vi "Arm Encoder.vi"(6 "Reset Encoder?":bool, 8 "Mode":enum16{"Init", "Run", "End"}(ring), 11 "Digital Module A":T1={"DIO Module"=enum."Digital Module 2", "Left Encoder B Channel"=enum."DIO 1", "Left Encoder A Channel"=enum."DIO 2", "Right Encoder B Channel"=enum."DIO 3", "Right Encoder A Channel"=enum."DIO 4", "Arm Encoder A Channel"=enum."DIO 5", "Arm Encoder B Channel"=enum."DIO 6", "Pressure Switch"=enum."DIO 7", "Unassigned"=enum."DIO 8", "Unassigned"=enum."DIO 9", "Ultrasonic Trigger"=enum."DIO 10", "Remus Switch"=enum."DIO 11", "Unassigned"=enum."DIO 12", "Unassigned"=enum."DIO 13", "Unassigned"=enum."DIO 14"}) -> (2 "Get Arm Encoder":dbl)   [LabVIEW 2013]
doc: "This example shows how to move a motor connected to an encoder and a wheel, and then read information about the system from an encoder.\n\nThis is an example of how to use feedback (from the encoder) to create an open loop system. If some control method was used, for example using PID, a closed loop system could be created."
uses:
  <vilib>/Rock Robotics/WPI/Encoder/WPI_EncoderType.ctl
  Type Defs/Digital Module A.ctl
  <vilib>/Rock Robotics/SystemInterfaces/Typedef/FPGA_TypedefDigitalModule.ctl
  <vilib>/Rock Robotics/SystemInterfaces/DIO/FPGA_DIOChannel.ctl
  <vilib>/Rock Robotics/WPI/Counter/WPI_CounterDigitalInputToDigitalSource.vi
panel:
  out "Arm Encoder Direction":string="Backward"
  in  "Decoding Type":T4=enum."4x"
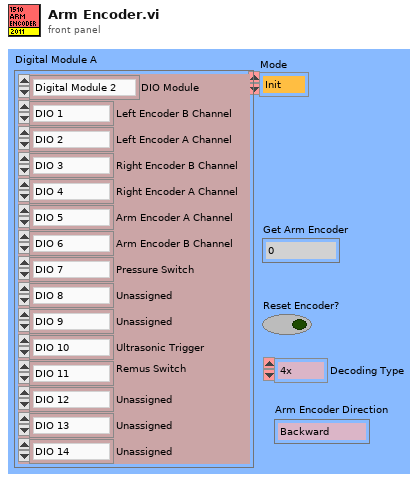
[diagram p1: front panel]
types:
  T1 = typedef "Digital Module A.ctl" = cluster{"DIO Module":T2, "Left Encoder B Channel":T3, "Left Encoder A Channel":T3, "Right Encoder B Channel":T3, "Right Encoder A Channel":T3, "Arm Encoder A Channel":T3, "Arm Encoder B Channel":T3, "Pressure Switch":T3, "Unassigned":T3, "Unassigned":T3, "Ultrasonic Trigger":T3, "Remus Switch":T3, "Unassigned":T3, "Unassigned":T3, "Unassigned":T3}
  T2 = typedef "FPGA_TypedefDigitalModule.ctl" = enum16{"Digital Module 1", "Digital Module 2"}
  T3 = typedef "FPGA_DIOChannel.ctl" = enum8{"DIO 1", "DIO 2", "DIO 3", "DIO 4", "DIO 5", "DIO 6", "DIO 7", "DIO 8", "DIO 9", "DIO 10", "DIO 11", "DIO 12", "DIO 13", "DIO 14", "Invalid"}
  T4 = typedef "WPI_EncoderType.ctl" = enum16{"1x", "2x", "4x"}
  T5 = typedef "WPI_DigitalInputDevRef.ctl" = cluster{"DevStatus":errorcluster, "DIO Channel":T3, "Digital Module":T2}
  T6 = typedef "FPGA_CounterEncoderSourceConvertionLVSourceType.ctl" = cluster{"DevStatus":errorcluster, "AnalogTriggerMode?":bool, "DigitalMode":cluster{"Digital Module":T2, "DIO Channel":T7}, "AnalogTriggerMode":cluster{"AnalogTriggerIndex":T8, "OutputType":T9}}
  T7 = typedef "FPGA_DIODigitalSourceChannel.ctl" = enum8{"DIO 1", "DIO 2", "DIO 3", "DIO 4", "DIO 5", "DIO 6", "DIO 7", "DIO 8", "DIO 9", "DIO 10", "DIO 11", "DIO 12", "DIO 13", "DIO 14", "Disabled"}
  T8 = typedef "FPGA_AnalogTriggerIndex.ctl" = enum8{"Trig 0", "Trig 1", "Trig 2", "Trig 3", "Trig 4", "Trig 5", "Trig 6", "Trig 7", "Invalid"}
  T9 = typedef "FPGA_AnalogTriggerOutType.ctl" = enum16{"InWindow", "TriggerState", "Rising", "Falling"}
  T10 = typedef "WPI_EncoderDevRef.ctl" = cluster{"DevStatus":errorcluster, "EncoderIndex":T11, "CounterIndex":T12, "DistancePerCount":dbl, "Decoding Type":T4}
  T11 = typedef "FPGA_EncoderIdx.ctl" = enum8{"Enc 0", "Enc 1", "Enc 2", "Enc 3", "Invalid"}
  T12 = typedef "FPGA_CounterCtrSystemIndex.ctl" = enum8{"Ctr 0", "Ctr 1", "Ctr 2", "Ctr 3", "Ctr 4", "Ctr 5", "Ctr 6", "Ctr 7", "Invalid"}
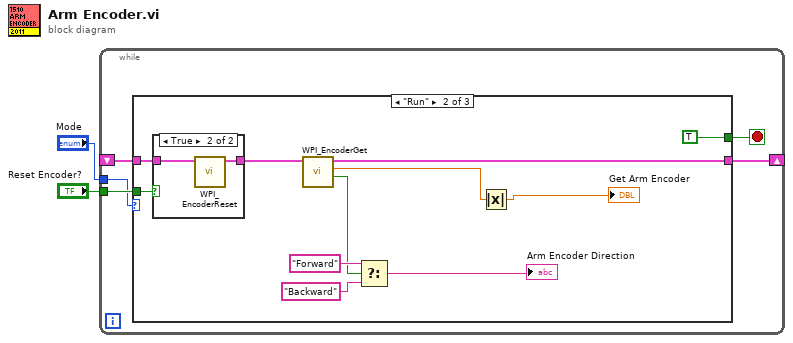
[diagram p0: block diagram]
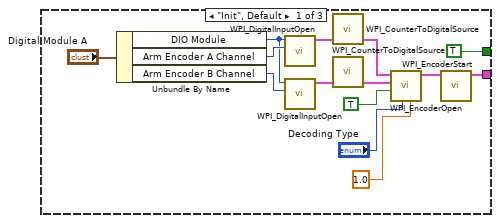
[diagram p2: hidden frame]
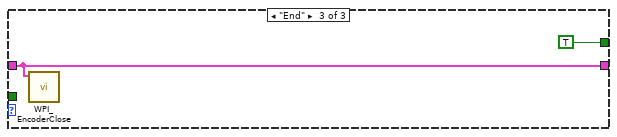
[diagram p4: hidden frame]
diagram:
  n1 = while {
    shift-right: [w6] -> _
    shift-left: _ -> [w5]
    tunnel: "Reset Encoder?" -> [w4]
    tunnel: "Mode" -> [w3]
    stop <- w7 stop-if-true
    n2 = case shown="\"Run\"" w3 {
      tunnel: [TRUE TRUE TRUE] -> w7
      tunnel: [w11 w26 w36] -> w6
      tunnel: w5 -> [_ w31 w36]
      tunnel: w4 -> [_ w24 _]
      frame "Init", Default {
        n3 = Unbundle By Name("Digital Module A") -> ("DIO Module"=w12:T2, "Arm Encoder A Channel"=w14:T3, "Arm Encoder B Channel"=w13:T3)
        n4 = call <vilib>:"WPI_DigitalInputOpen.vi"("DIO Channel"=w14, "Digital Module (Module 1)"=w12) -> ("DigitalInputDevRef"=w18:T5)  [unwired: 1 in, 8 out]
        n5 = call <vilib>:"WPI_DigitalInputOpen.vi"("DIO Channel"=w13, "Digital Module (Module 1)"=w12) -> ("DigitalInputDevRef"=w19:T5)  [unwired: 1 in, 8 out]
        n6 = call-poly <vilib>:"WPI_CounterToDigitalSource.vi"("DigitalInputDevRef"=w18) -> ("Digital Source"=w17:T6)  [unwired: 1 in, 5 out]
        n7 = call-poly <vilib>:"WPI_CounterToDigitalSource.vi"("DigitalInputDevRef"=w19) -> ("Digital Source"=w16:T6)  [unwired: 6 out]
        n8 = call <vilib>:"WPI_EncoderOpen.vi"("DistancePerCount"=1.0, "Decoding Type"="Decoding Type", "Invert Direction (False)"=TRUE, "BSource"=w16, "ASource"=w17) -> ("EncoderDevRef"=w9:T10)  [unwired: 3 in, 3 out]
        n9 = call <vilib>:"WPI_EncoderStart.vi"("EncoderDevRef"=w9) -> ("EncoderDevRef"=w11:T10)  [unwired: 1 in, 9 out]
      }
      frame "Run" {
        n10 = case shown="True" w24 {
          tunnel: w31 -> [w33 w35]
          tunnel: [w33 w34] -> w25
          frame False {
          }
          frame True {
            n11 = call <vilib>:"WPI_EncoderReset.vi"("EncoderDevRef"=w35) -> ("EncoderDevRef"=w34:T10)  [unwired: 1 in, 9 out]
          }
        }
        n12 = call <vilib>:"WPI_EncoderGet.vi"("EncoderDevRef"=w25) -> ("Direction"=w27:bool, "Distance"=w23:dbl, "EncoderDevRef"=w26:T10)  [unwired: 1 in, 7 out]
        n13 = Select(t="Forward", s=w27, f="Backward") -> (s? t:f=→"Arm Encoder Direction":string)
        n14 = Absolute Value(x=w23) -> (abs(x)=→"Get Arm Encoder":dbl)
      }
      frame "End" {
        n15 = call <vilib>:"WPI_EncoderClose.vi"("EncoderDevRef"=w36) -> ()  [unwired: 2 in, 9 out]
      }
    }
  }
